vi "Energy and amplitude panel.vi"() -> ()   [LabVIEW 2017]
uses:
  control panel globals.vi
  <vilib>/Analysis/NI_AALPro.lvlib
panel:
  out "major axis":dbl format="%#.1f"
  in  "take snapshot":bool
  out "maj axis sq.":sgl
  out "amplitude sq lifetime":dbl
  in  "clear slope and mag data":bool
  out "maj axis vs time":cluster{dbl[], dbl[]}[](graph)
  out "slope vs maj axis":cluster{dbl[], "Best Polynomial Fit":dbl[]}[](graph)
  out "error out":errorcluster
  in  "log slope and maj axis?":bool
  in  "fit last _ seconds":dbl=5000.0
  out "Q":dbl
  out "slope":dbl
  out "slope lifetime":dbl
  out "slope vs time":cluster{dbl[], dbl[]}[](graph)
  # "omega tau!"
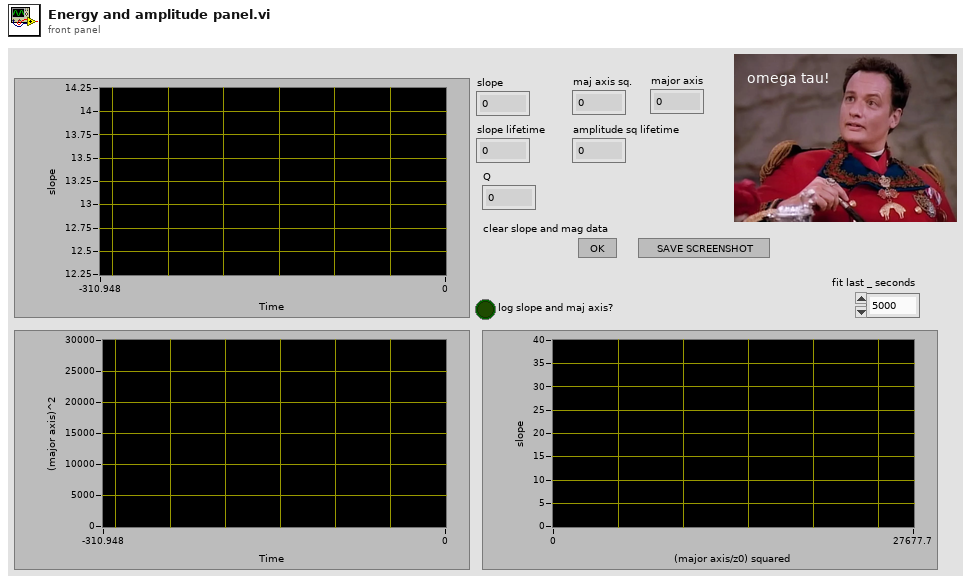
[diagram p1: front panel]
types:
  T1 = typedef "queue cluster.ctl" = cluster{"voltage":T2, "coil":T2, "mag":refnum<queue>, "accel":T2, "crossing":T2, "orbit fit":refnum<queue>, "pulse":T2, "mag0":T2, "fitLocation":refnum<queue>}
  T2 = typedef "reading queue.ctl" = refnum<queue>
  T3 = typedef "orbit parameters with crossing info.ctl" = cluster{"a":dbl, "b":dbl, "theta_axis":dbl, "dPhi":dbl, "BrV":dbl, "bob tilt":dbl, "phi0":dbl, "phi_dot":dbl, "x0":dbl, "y0":dbl, "z0":dbl, "mid crossing time":dbl, "most recent crossing number":dbl, "most recent crossing slope":dbl, "most recent crossing period":dbl}
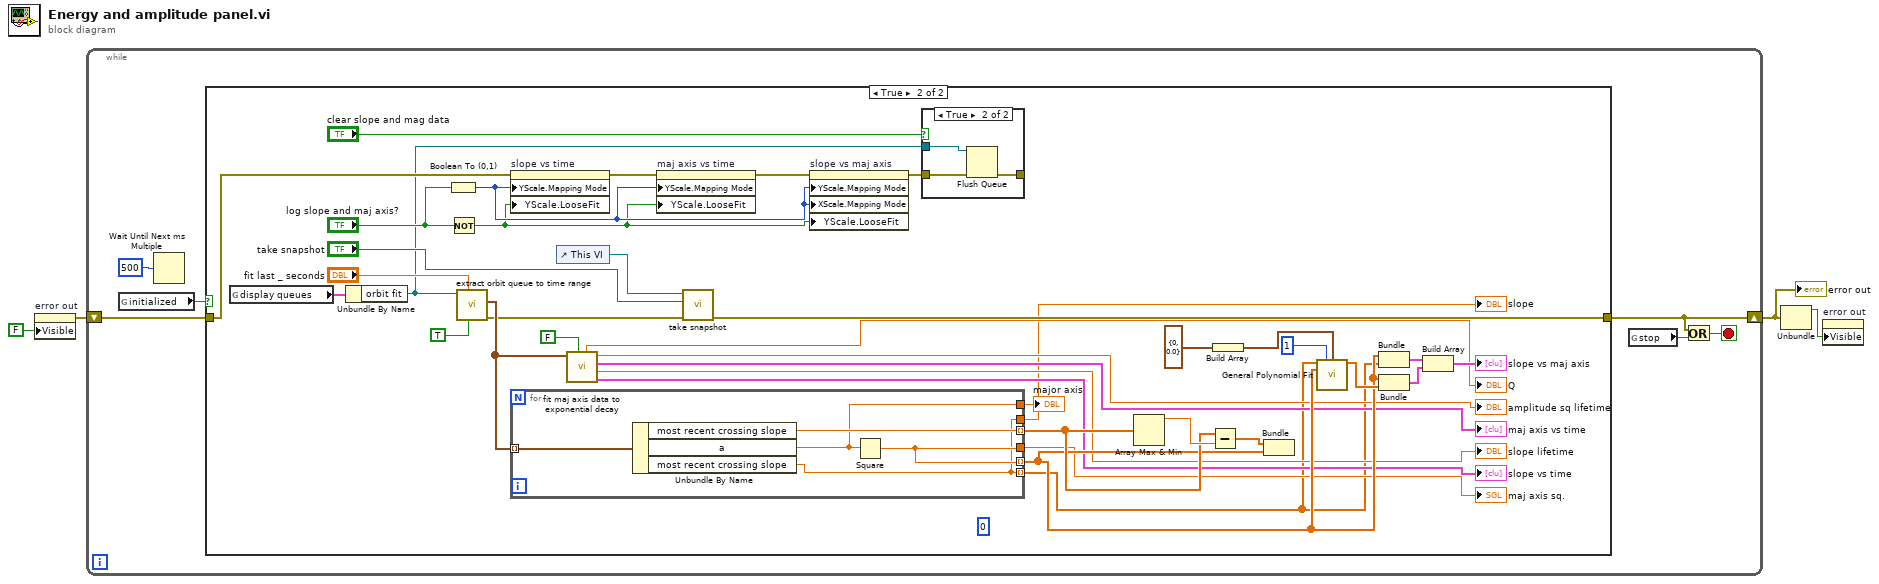
[diagram p0: block diagram]
diagram:
  n1 = property on="error out" class="Clust (strict)"("Visible"=FALSE) -> (error out=w4:errorcluster)  [unwired: 2 in, 1 out]
  n2 = while {
    shift-right: [w8] -> w2
    shift-left: w4 -> [w9]
    stop <- w7 stop-if-true
    n3 = global read "control panel globals.vi" "initialized"() -> (w10:bool)
    n4 = Wait Until Next ms Multiple(millisecond multiple=u32 500) -> ()  [unwired: 1 out]
    n5 = case shown="True" w10 {
      tunnel: [w11 w20] -> w8
      tunnel: w9 -> [w11 w48]
      frame False {
      }
      frame True {
        (unwired) 0 ("index")
        n6 = global read "control panel globals.vi" "display queues"() -> (w49:T1)
        n7 = Unbundle By Name(w49) -> ("orbit fit"=w18:refnum<queue>)
        n8 = Boolean To (0,1)(Boolean="log slope and maj axis?") -> (0, 1=w42:i16)
        n9 = Not(x="log slope and maj axis?") -> (.not. x?=w35:bool)
        n10 = call "extract orbit queue to time range.vi"("most recent?"=TRUE, "recent interval"="fit last _ seconds", "orbit fit"=w18) -> ("error out"=w21:errorcluster, "extracted elements"=w29:T3[])  [unwired: 7 in]
        n11 = property on="slope vs time" class="XYGraph (strict)"(error in=w48, "YScale.Mapping Mode"=w42, "YScale.LooseFit"=w35) -> (error out=w41:errorcluster)  [unwired: 1 in, 1 out]
        n12 = for {
          tunnel: w29 -> [w57] mode=indexing
          tunnel: [w56] -> w30 mode=indexing
          tunnel: [w58] -> w44 mode=indexing
          tunnel: [w56] -> w23
          tunnel: [w55] -> w14 mode=indexing
          tunnel: [w55] -> w13
          tunnel: [w54] -> w12
          n13 = Unbundle By Name(w57) -> ("most recent crossing slope"=w58:dbl, "a"=w54:dbl, "most recent crossing slope"=w55:dbl)
          n14 = Square(x=w54) -> (x^2=w56:dbl)
        }
        "slope" <- w13
        "maj axis sq." <- w23
        "major axis" <- w12
        n15 = control-ref of="This VI"() -> (w22:refnum<vi>)
        n16 = call "fit maj axis data to exponential decay.vi"("hrs"=FALSE, "extracted data"=w29) -> ("slope graphs"=→"slope vs time":cluster{dbl[], dbl[]}[], "slope lifetime"=→"slope lifetime":dbl, "graphs"=→"maj axis vs time":cluster{dbl[], dbl[]}[], "lifetime"=→"amplitude sq lifetime":dbl, "Q"=→"Q":dbl)  [unwired: 4 in, 1 out]
        n17 = property on="maj axis vs time" class="XYGraph (strict)"(error in=w41, "YScale.Mapping Mode"=w42, "YScale.LooseFit"=w35) -> (error out=w40:errorcluster)  [unwired: 1 in, 1 out]
        n18 = call "take snapshot.vi"("error in (no error)"=w21, "take snapshot"="take snapshot", "vi ref"=w22) -> ("error out"=w20:errorcluster)  [unwired: 8 in]
        n19 = property on="slope vs maj axis" class="XYGraph (strict)"(error in=w40, "YScale.Mapping Mode"=w42, "XScale.Mapping Mode"=w42, "YScale.LooseFit"=w35) -> (error out=w37:errorcluster)  [unwired: 1 in, 1 out]
        n20 = case shown="True" "clear slope and mag data" {
          tunnel: w37 -> [w50 w53]
          tunnel: [w50 w52] -> _
          tunnel: w18 -> [_ w51]
          frame False {
          }
          frame True {
            n21 = Flush Queue(queue=w51, error in (no error)=w53) -> (error out=w52:errorcluster)  [unwired: 2 out]
          }
        }
        n22 = Array Max & Min(array=w44) -> (max value=w46:dbl)  [unwired: 3 out]
        n23 = Subtract(x=w44, y=w46) -> (x-y=w45:dbl[])
        n24 = Build Array(cluster{"order":i32, "coefficient":dbl} {"order"=0, "coefficient"=0.0} ("Cluster")) -> (w24:cluster{"order":i32, "coefficient":dbl}[])
        n25 = Bundle(w45, w30) -> ()  [unwired: 1 in, 1 out]
        n26 = call <vilib>:"General Polynomial Fit.vi"("Y"=w14, "polynomial order"=1, "Coefficient Constraint"=w24, "X"=w30) -> ("Best Polynomial Fit"=w31:dbl[])  [unwired: 8 in, 3 out]
        n27 = Bundle(w30, w14) -> (w43:cluster{dbl[], dbl[]})  [unwired: 1 in]
        n28 = Bundle(w30, "Best Polynomial Fit"=w31) -> (w32:cluster{dbl[], "Best Polynomial Fit":dbl[]})  [unwired: 1 in]
        n29 = Build Array(w43, w32) -> (→"slope vs maj axis":cluster{dbl[], "Best Polynomial Fit":dbl[]}[])
      }
    }
    n30 = global read "control panel globals.vi" "stop"() -> (w6:bool)
    n31 = Or(x=w8, y=w6) -> (x .or. y?=w7:bool)
  }
  "error out" <- w2
  n32 = Unbundle(w2) -> ("status"=w1:bool)  [unwired: 2 out]
  n33 = property on="error out" class="Clust (strict)"("Visible"=w1) -> ()  [unwired: 2 in, 2 out]
